vi "daqReadEtl.vi"() -> ()   [LabVIEW 2017]
doc: "From the DAQ card, reads into shared variables the external frame counter, the piezo monitor, and its differentiator. The acquisition is triggered by the Hamamatsu camera triggers. If daqSave is set to true, writes the values to file. \n\nThe acquisition loop stops with a daqStop (generally issued by the hamamatsuRead* VI) or, after a delay, with a generalStop."
uses:
  <vilib>/DAQmx/read.llb/DAQmx Read (Analog 1D DBL NChan 1Samp).vi
  <vilib>/DAQmx/read.llb/DAQmx Read (Counter U32 1Chan 1Samp).vi
  globalDevices.vi
  globalUtilities.vi
  <vilib>/DAQmx/miscellaneous.llb/DAQmx Fill In Error Info.vi
panel:
  out "x+y":u32
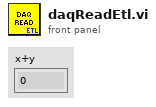
[diagram p1: front panel]
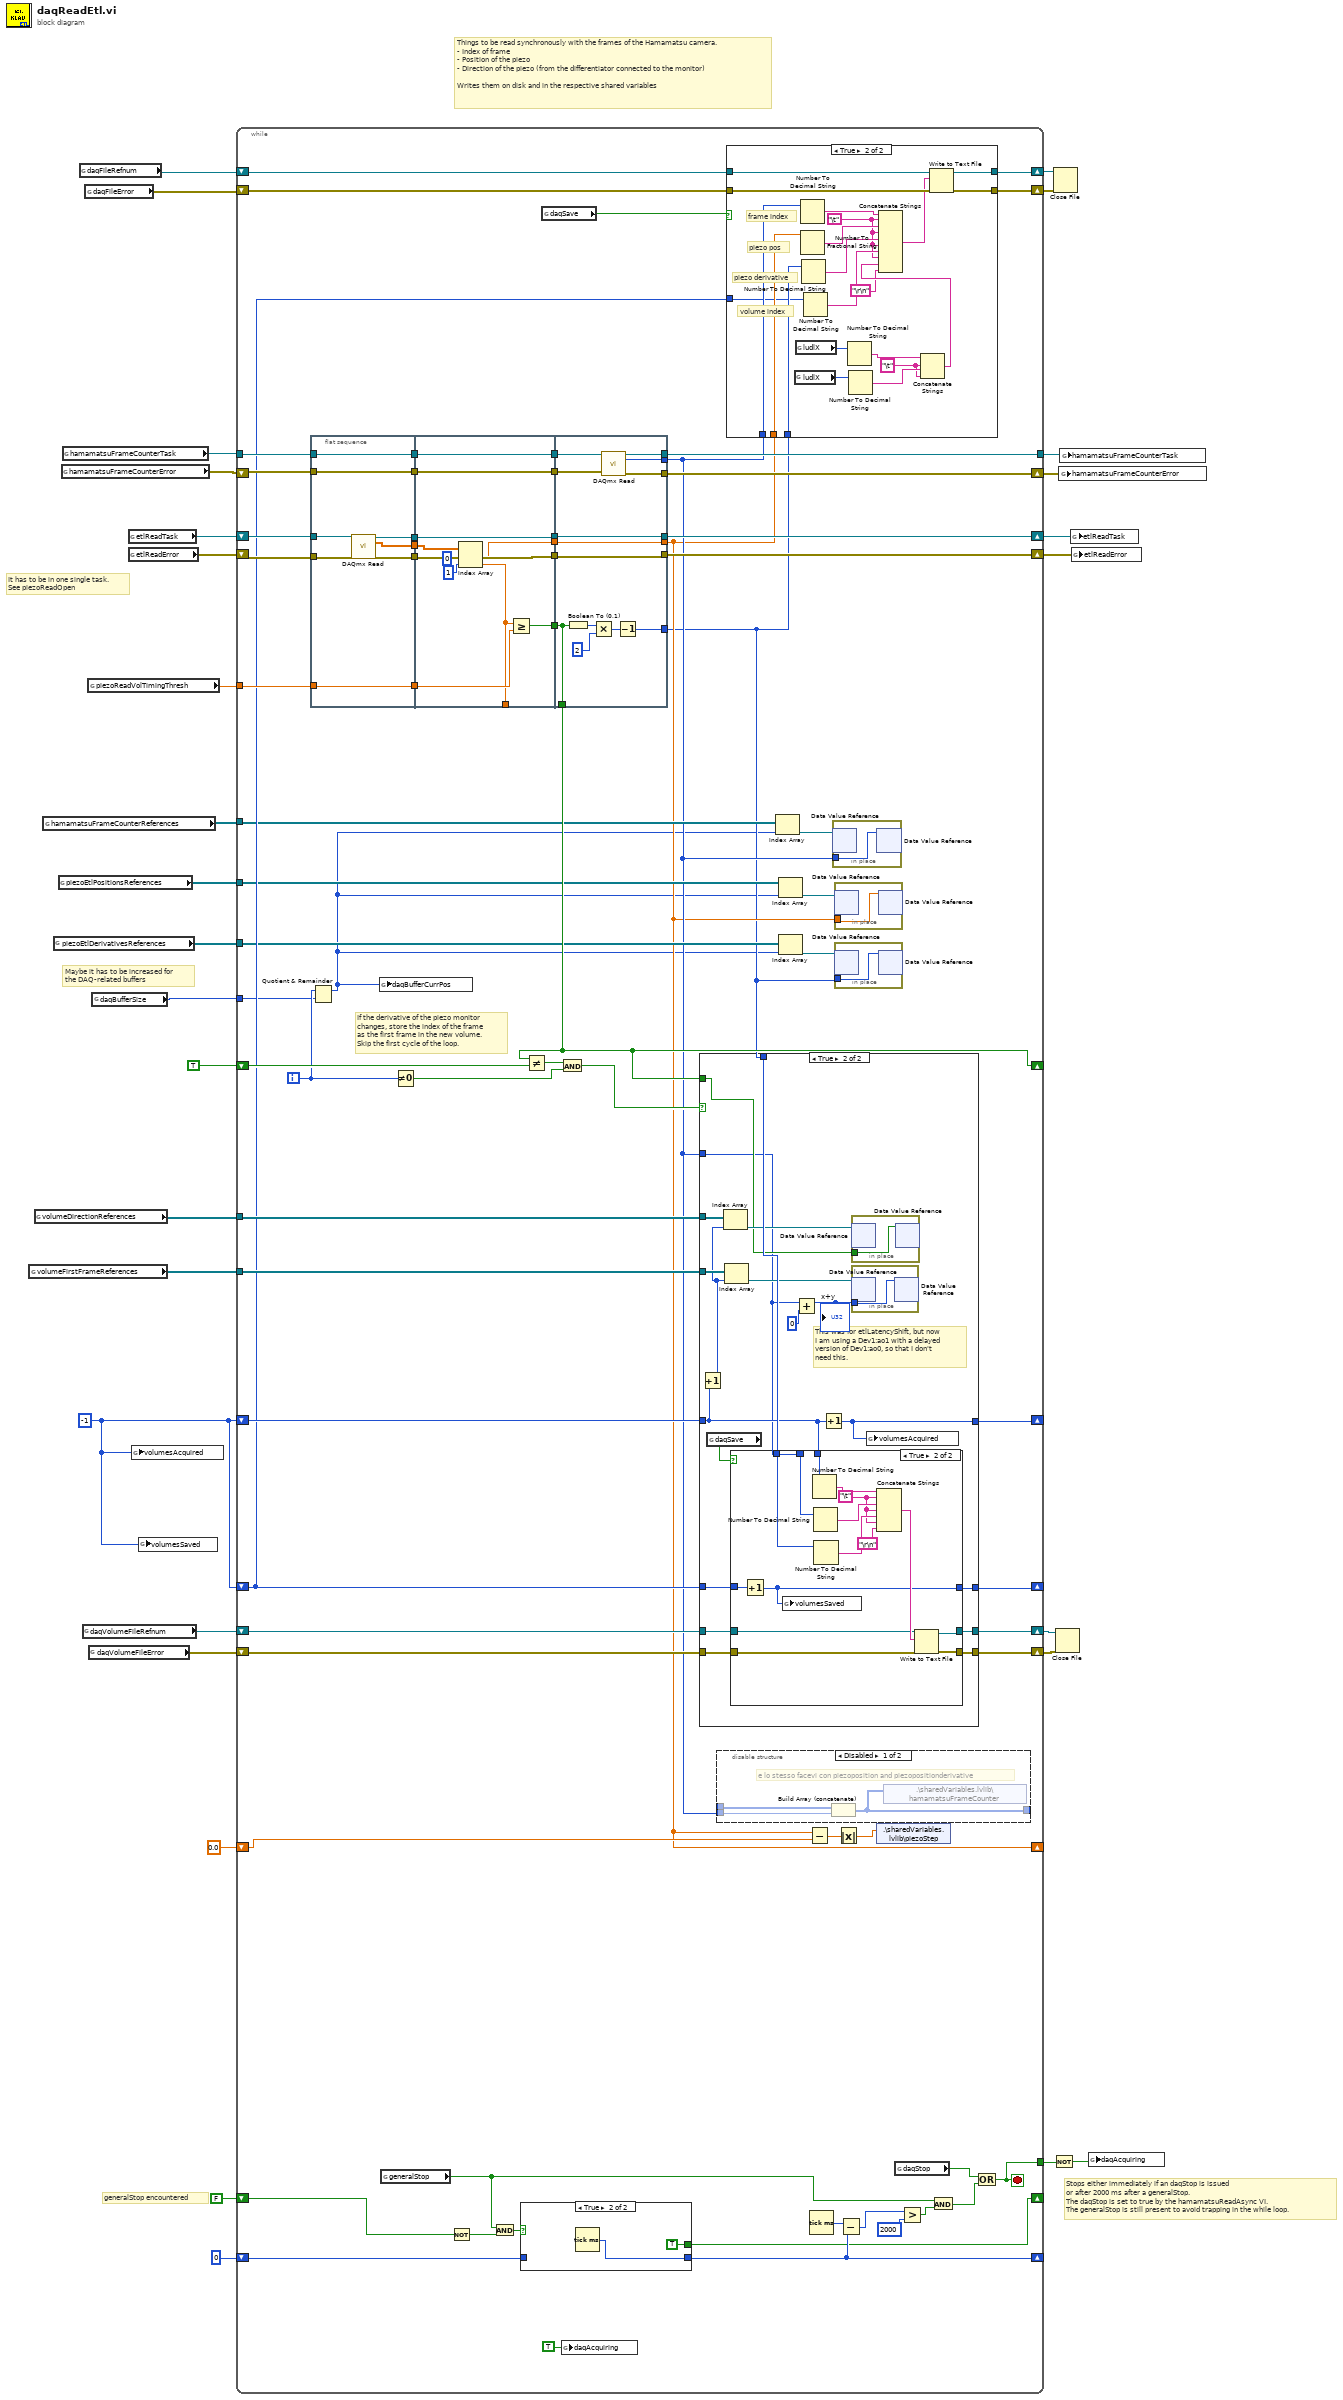
[diagram p0: block diagram]
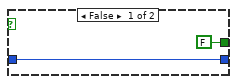
[diagram p5: hidden frame]
diagram:
  w7 = -1
  # "Maybe it has to be increased for\nthe DAQ-related buffers"
  # "It has to be in one single task.\nSee piezoReadOpen"
  # "generalStop encountered"
  # "Stops either immediately if an daqStop is issued\nor after 2000 ms after a generalStop.\nThe daqStop is set to true by the hamamatsuReadAsync VI.\nThe generalStop is still present to avoid trapping in the while loop."
  # "Things to be read synchronously with the frames of the Hamamatsu camera.\n- Index of frame\n- Position of the piezo\n- Direction of the piezo (from the differentiator connected to the monitor)\n\nWrites them on disk and in the respective shared variables"
  n1 = global read "globalUtilities.vi" "volumeFirstFrameReferences"() -> (w8:refnum<data-value>[])
  n2 = global read "globalUtilities.vi" "volumeDirectionReferences"() -> (w9:refnum<data-value>[])
  n3 = global read "globalDevices.vi" "hamamatsuFrameCounterReferences"() -> (w4:refnum<data-value>[])
  n4 = global read "globalDevices.vi" "piezoEtlDerivativesReferences"() -> (w2:refnum<data-value>[])
  n5 = global read "globalDevices.vi" "piezoEtlPositionsReferences"() -> (w3:refnum<data-value>[])
  n6 = global read "globalDevices.vi" "hamamatsuFrameCounterError"() -> (w29:errorcluster)
  n7 = global read "globalDevices.vi" "hamamatsuFrameCounterTask"() -> (w30:refnum<k21>)
  n8 = global read "globalDevices.vi" "daqFileRefnum"() -> (w19:refnum<file>)
  n9 = global read "globalDevices.vi" "daqVolumeFileRefnum"() -> (w13:refnum<file>)
  n10 = global read "globalDevices.vi" "daqFileError"() -> (w18:errorcluster)
  n11 = global read "globalDevices.vi" "piezoReadVolTimingThresh"() -> (w25:dbl)
  n12 = global read "globalDevices.vi" "daqVolumeFileError"() -> (w12:errorcluster)
  n13 = global read "globalDevices.vi" "daqBufferSize"() -> (w1:i32)
  n14 = global read "globalDevices.vi" "etlReadTask"() -> (w6:refnum<k21>)
  n15 = global read "globalDevices.vi" "etlReadError"() -> (w5:errorcluster)
  n16 = global write "globalUtilities.vi" "volumesAcquired"(w7) -> ()
  n17 = global write "globalUtilities.vi" "volumesSaved"(w7) -> ()
  n18 = while {
    tunnel: w30 -> [w99]
    shift-right: [w95] -> w21
    shift-left: w29 -> [w97]
    shift-right: [w93] -> w22
    shift-left: w5 -> [w96]
    shift-right: [w90] -> w28
    shift-left: w19 -> [w91]
    shift-right: [w77] -> _
    shift-left: FALSE -> [w88]
    shift-right: [w82] -> _
    shift-left: u32 0 -> [w85]
    tunnel: w25 -> [w76]
    shift-right: [w56] -> _
    shift-left: TRUE -> [w74]
    shift-right: [w69] -> w23
    shift-left: w6 -> [w101]
    tunnel: [w68] -> w20
    shift-right: [w60] -> w17
    shift-left: w18 -> [w92]
    tunnel: [w57] -> w16
    shift-right: [w33] -> _
    shift-left: 0.0 -> [w55]
    shift-right: [w49] -> w10
    shift-left: w12 -> [w51]
    shift-right: [w50] -> w11
    shift-left: w13 -> [w52]
    shift-right: [w47] -> _
    shift-left: w7 -> [w48]
    tunnel: w9 -> [w46]
    tunnel: w8 -> [w45]
    shift-right: [w44] -> _
    shift-left: w7 -> [w43]
    tunnel: w4 -> [w42]
    tunnel: w3 -> [w41]
    tunnel: w2 -> [w40]
    tunnel: w1 -> [w38]
    i -> [w39]
    stop <- w57 stop-if-true
    # "If the derivative of the piezo monitor\nchanges, store the index of the frame\nas the first frame in the new volume.\nSkip the first cycle of the loop."
    n19 = flat-sequence {
      tunnel: w76 -> [w183]
      tunnel: w97 -> [w184]
      tunnel: w96 -> [w181]
      tunnel: w99 -> [w185]
      tunnel: w101 -> [w182]
      tunnel: [w185] -> w67
      tunnel: [w184] -> w66
      tunnel: [w183] -> w65
      tunnel: [w180] -> w64
      tunnel: [w179] -> w63
      tunnel: [w178] -> w61
      tunnel: [w196] -> w100
      tunnel: [w195] -> w98
      tunnel: [w191] -> w94
      tunnel: [w193] -> w75
      tunnel: [w186] -> _
      tunnel: [w192] -> w70
      tunnel: w67 -> [w196]
      tunnel: w66 -> [w195]
      tunnel: w65 -> [w194]
      tunnel: w64 -> [w192]
      tunnel: w63 -> [w190]
      tunnel: [w187] -> w62
      tunnel: w61 -> [w191]
      tunnel: w100 -> [w209]
      tunnel: w98 -> [w208]
      tunnel: [w207] -> w33
      tunnel: [w206] -> w34
      tunnel: [w205] -> w95
      tunnel: [w204] -> w93
      tunnel: w94 -> [w204]
      tunnel: w75 -> [w199]
      tunnel: [w200] -> w32
      tunnel: [w199] -> w56
      tunnel: w70 -> [w198]
      tunnel: [w198] -> w69
      tunnel: [w197] -> w68
      tunnel: w62 -> [w207]
      frame #0 {
        n20 = call-poly <vilib>:"DAQmx Read.vi"("task/channels in"=w182, "error in"=w181) -> ("task out"=w180:refnum<k21>, "data"=w179:dbl[], "error out"=w178:errorcluster)  [unwired: 11 in]
      }
      frame #1 {
        n21 = Index Array(array=w190, index #1=0 ("index"), index #2=1 ("index")) -> (element #1=w187:dbl, element #2=w186:dbl)
        n22 = Greater Or Equal?(x=w186, y=w194) -> (x >= y?=w193:bool)
      }
      frame #2 {
        n23 = Boolean To (0,1)(Boolean=w199) -> (0, 1=w203:i16)
        n24 = Multiply(x=w203, y=i16 2) -> (x*y=w201:i16)
        n25 = call-poly <vilib>:"DAQmx Read.vi"("task/channels in"=w209, "error in"=w208) -> ("task out"=w197:refnum<k21>, "data"=w206:u32, "error out"=w205:errorcluster)  [unwired: 11 in]
        n26 = Decrement(x=w201) -> (x-1=w200:i16)
      }
    }
    n27 = Quotient & Remainder(x=w39, y=w38) -> (x-y*floor(x/y)=w31:i32)  [unwired: 1 out]
    n28 = global write "globalDevices.vi" "daqBufferCurrPos"(w31) -> ()
    n29 = global read "globalUtilities.vi" "generalStop"() -> (w84:bool)
    n30 = Not Equal To 0?(x=w39) -> (x != 0?=w72:bool)
    n31 = Not(x=w88) -> (.not. x?=w86:bool)
    n32 = And(x=w84, y=w86) -> (x .and. y?=w87:bool)
    n33 = case shown="True" w87 {
      tunnel: w85 -> [w152 _]
      tunnel: [w152 w154] -> w82
      tunnel: [FALSE TRUE] -> w77
      frame False {
      }
      frame True {
        n34 = Tick Count (ms)() -> (millisecond timer value=w154:u32)
      }
    }
    n35 = Not Equal?(x=w56, y=w74) -> (x != y?=w73:bool)
    n36 = global read "globalUtilities.vi" "daqSave"() -> (w89:bool)
    n37 = And(x=w73, y=w72) -> (x .and. y?=w71:bool)
    n38 = global write "globalUtilities.vi" "daqAcquiring"(TRUE ("daqAcquiring")) -> ()
    n39 = case shown="True" w71 {
      tunnel: w34 -> [_ w117]
      tunnel: w56 -> [_ w121]
      tunnel: w52 -> [w110 w129]
      tunnel: w51 -> [w109 w128]
      tunnel: [w110 w127] -> w50
      tunnel: [w109 w126] -> w49
      tunnel: w48 -> [w111 w119]
      tunnel: [w111 w124] -> w47
      tunnel: w32 -> [_ w125]
      tunnel: w46 -> [_ w123]
      tunnel: w45 -> [_ w120]
      tunnel: w43 -> [w108 w115]
      tunnel: [w108 w114] -> w44
      frame False {
      }
      frame True {
        # "This was for etlLatencyShift, but now\nI am using a Dev1:ao1 with a delayed \nversion of Dev1:ao0, so that I don't \nneed this."
        n40 = Increment(x=w119) -> (x+1=w116:i32)
        n41 = global read "globalUtilities.vi" "daqSave"() -> (w130:bool)
        n42 = Index Array(array=w123, index=w116) -> (element=w122:refnum<data-value>)
        n43 = Index Array(array=w120, index=w116) -> (element=w118:refnum<data-value>)
        n44 = case shown="True" w130 {
          tunnel: w129 -> [w135 w141]
          tunnel: w128 -> [w134 w140]
          tunnel: [w135 w139] -> w127
          tunnel: [w134 w138] -> w126
          tunnel: w119 -> [_ w150]
          tunnel: w117 -> [_ w149]
          tunnel: w125 -> [_ w148]
          tunnel: w115 -> [w133 w137]
          tunnel: [w133 w136] -> w114
          frame False {
          }
          frame True {
            w144 = "\t"
            n45 = Increment(x=w137) -> (x+1=w136:i32)
            n46 = global write "globalUtilities.vi" "volumesSaved"(w136) -> ()
            n47 = Number To Decimal String(number=w150) -> (decimal integer string=w147:string)  [unwired: 1 in]
            n48 = Number To Decimal String(number=w149) -> (decimal integer string=w146:string)  [unwired: 1 in]
            n49 = Number To Decimal String(number=w148) -> (decimal integer string=w145:string)  [unwired: 1 in]
            n50 = Concatenate Strings(w147, w144, w146, w144, w145, w144, "\r\n") -> (w142:string)
            n51 = Write to Text File(file (use dialog)=w141, text=w142, error in=w140) -> (refnum out=w139:refnum<file>, error out=w138:errorcluster)  [unwired: 1 in, 1 out]
          }
        }
        n52 = Add(x=w117, y=u32 0) -> (x+y=w113:u32)
        "x+y" <- w113
        n53 = Increment(x=w119) -> (x+1=w124:i32)
        n54 = in-place {
          in-place-border: w121 -> [w132]
          n55 = in-place-dvr #1(w122) -> ()  [unwired: 2 out]
          n56 = in-place-dvr #1(w132) -> ()  [unwired: 2 out]
        }
        n57 = in-place {
          in-place-border: w113 -> [w131]
          n58 = in-place-dvr #2(w118) -> ()  [unwired: 2 out]
          n59 = in-place-dvr #2(w131) -> ()  [unwired: 2 out]
        }
        n60 = global write "globalUtilities.vi" "volumesAcquired"(w124) -> ()
      }
    }
    n61 = disable-structure shown="Disabled" {
      disable-tunnel: _ -> [w104 _]
      disable-tunnel: [w103 _] -> _
      disable-tunnel: w34 -> [w102 _]
      frame Disabled {
        # "e lo stesso facevi con piezoposition and piezopositionderivative"
        n62 = Build Array (concatenate)(w104, w102) -> (w103:u32[])
        n63 = shared-variable ".\\sharedVariables.lvlib\\hamamatsuFrameCounter"(w103) -> ()  [unwired: 1 in, 1 out]
      }
      frame Enabled {
      }
    }
    n64 = case shown="True" w89 {
      tunnel: w92 -> [w155 w175]
      tunnel: w91 -> [w156 w173]
      tunnel: [w156 w172] -> w90
      tunnel: [w155 w171] -> w60
      tunnel: w34 -> [_ w170]
      tunnel: w33 -> [_ w169]
      tunnel: w32 -> [_ w167]
      tunnel: w43 -> [_ w166]
      frame False {
      }
      frame True {
        w160 = "\t" ("string")
        w159 = "\t"
        # "volume index"
        # "piezo derivative"
        # "piezo pos"
        # "frame index"
        n65 = global read "globalDevices.vi" "ludlX"() -> (w161:i32)
        n66 = global read "globalDevices.vi" "ludlX"() -> (w162:i32)
        n67 = Number To Decimal String(number=w170) -> (decimal integer string=w177:string)  [unwired: 1 in]
        n68 = Number To Fractional String(number=w169) -> (F-format string=w176:string)  [unwired: 3 in]
        n69 = Number To Decimal String(number=w167) -> (decimal integer string=w168:string)  [unwired: 1 in]
        n70 = Number To Decimal String(number=w166) -> (decimal integer string=w165:string)  [unwired: 1 in]
        n71 = Number To Decimal String(number=w162) -> (decimal integer string=w163:string)  [unwired: 1 in]
        n72 = Number To Decimal String(number=w161) -> (decimal integer string=w164:string)  [unwired: 1 in]
        n73 = Concatenate Strings(w163, w160, w164, w160) -> (w158:string)
        n74 = Concatenate Strings(w177, w159, w176, w159, w168, w159, w165, w159, w158, "\r\n") -> (w174:string)
        n75 = Write to Text File(file (use dialog)=w173, text=w174, error in=w175) -> (refnum out=w172:refnum<file>, error out=w171:errorcluster)  [unwired: 1 in, 1 out]
      }
    }
    n76 = Index Array(array=w42, index=w31) -> (element=w37:refnum<data-value>)
    n77 = Index Array(array=w41, index=w31) -> (element=w36:refnum<data-value>)
    n78 = Index Array(array=w40, index=w31) -> (element=w35:refnum<data-value>)
    n79 = Subtract(x=w33, y=w55) -> (x-y=w54:dbl)
    n80 = Tick Count (ms)() -> (millisecond timer value=w83:u32)
    n81 = in-place {
      in-place-border: w34 -> [w107]
      n82 = in-place-dvr #3(w37) -> ()  [unwired: 2 out]
      n83 = in-place-dvr #3(w107) -> ()  [unwired: 2 out]
    }
    n84 = in-place {
      in-place-border: w33 -> [w106]
      n85 = in-place-dvr #4(w36) -> ()  [unwired: 2 out]
      n86 = in-place-dvr #4(w106) -> ()  [unwired: 2 out]
    }
    n87 = in-place {
      in-place-border: w32 -> [w105]
      n88 = in-place-dvr #5(w35) -> ()  [unwired: 2 out]
      n89 = in-place-dvr #5(w105) -> ()  [unwired: 2 out]
    }
    n90 = Absolute Value(x=w54) -> (abs(x)=w53:dbl)
    n91 = Subtract(x=w83, y=w82) -> (x-y=w81:u32)
    n92 = shared-variable ".\\sharedVariables.lvlib\\piezoStep"(w53) -> ()  [unwired: 1 in, 1 out]
    n93 = global read "globalUtilities.vi" "daqStop"() -> (w58:bool)
    n94 = Greater?(x=w81, y=u32 2000) -> (0:w79:bool)
    n95 = And(x=w84, y=w79) -> (x .and. y?=w78:bool)
    n96 = Or(x=w58, y=w78) -> (x .or. y?=w57:bool)
  }
  n97 = Not(x=w16) -> (.not. x?=w15:bool)
  n98 = Close File(refnum=w28, error in=w17) -> ()  [unwired: 2 out]
  n99 = Close File(refnum=w11, error in=w10) -> ()  [unwired: 2 out]
  n100 = global write "globalDevices.vi" "hamamatsuFrameCounterError"(w21) -> ()
  n101 = global write "globalDevices.vi" "hamamatsuFrameCounterTask"(w20) -> ()
  n102 = global write "globalDevices.vi" "etlReadTask"(w23) -> ()
  n103 = global write "globalDevices.vi" "etlReadError"(w22) -> ()
  n104 = global write "globalUtilities.vi" "daqAcquiring"(w15) -> ()
